vi "Step_Delay_Tommaso_fixed_EPICS.vi"() -> ()   [LabVIEW 2019]
uses:
  <vilib>/DAQmx/write.llb/DAQmx Write (Analog DBL 1Chan 1Samp).vi
  <vilib>/DAQmx/miscellaneous.llb/DAQmx Fill In Error Info.vi
  <vilib>/DAQmx/create/channels.llb/DAQmx Create Channel (AO-Voltage-Basic).vi
  <userlib>/caLab/Private/Put_Boolean-1D_PV.vi
  <vilib>/Analysis/1siggen.llb/Ramp Pattern by Delta.vi
  <userlib>/caLab/Private/Put_Boolean-1D_PV-1D.vi
  Driver/Newport ESP301/Newport ESP301.lvlib
  <vilib>/Analysis/NI_AALBase.lvlib
panel:
  out "IOC started":bool=TRUE
  in  "Config File":path=path "T:/trARPES/Labview/Front ends/METIS_delayscan/delayScanEPICS.conf" caption="Soft IOC configuration file"
  in  "Configuration Set":T1(array[cluster])=[{"PV name"="trARPES:DelayStage:t0", "description"="Delay Stage time zero Position", "data type"="ai", "number of elements (waveform only)"=1, "element size (waveform only)"="", []}, {"PV name"="trARPES:DelayStage:p1", "description"="Delay Stage range start", "data type"="ai", "number of elements (waveform only)"=1, "element size (waveform only)"="", []}, {"PV name"="trARPES:DelayStage:p2", "description"="Delay Stage range end", "data type"="ai", "number of elements (waveform only)"=1, "element size (waveform only)"="", []}, {"PV name"="trARPES:DelayStage:Pos", "description"="Current Delay Stage position", "data type"="ai", "number of elements (waveform only)"=1, "element size (waveform only)"="", []}]
  in  "Dwell_positions":string[][](table)=[["-500", "3000"], ["-100", "3000"], ["0", "5000"], ["100", "5000"], ["500", "5000"], ["750", "10000"], ["1000", "10000"], ["", ""]]
  in  "Enable2":bool caption="Enable?"
  in  "Wait time [ms]":u32=1000 caption="Values <50 \nwon't work"
  out "StepSize [mm]":dbl=0.14989622900000002
  in  "stop 2":bool
  in  "StepSize [fs]":i32=1000
  in  "Enable?":bool
  out "a":waveform(dbl)(graph)={"t0"=timestamp(3675940489.011235 s since 1904-01-01), "dt"=1.0, "Y"=[-33.8895]}
  out "Waveform Chart":dbl(graph)=5.25341140860948
  out "x*y":dbl=-876.4751437142558
  in  "physical channels":tag="Dev1/ao1"
  out "DAC error":errorcluster
  out "ESP error":errorcluster
  out "run?":bool
  in  "set_vel":bool
  in  "velocity [fs/s]":dbl=333.564095198152
  in  "vel_mm":dbl=0.005 caption="velocity [mm/s]"
  out "meas. velocity":dbl
  in  "stop":bool
  out "output voltage":dbl
  in  "start":bool
  in  "go2p1":bool
  out "position [mm]":dbl=-33.8895
  in  "p2 [mm]":dbl=-0.707153771
  in  "p1 [mm]":dbl=-1.006946229
  in  "interpolate output":bool
  in  "Delta2 [fs]":dbl=999.9999999999999
  in  "Delta1 [fs]":dbl=-999.9999999999999
  in  "Reference [mm]":dbl=-0.85705
  in  "Axis (1)":i32=3 min=1 max=3
  in  "Serial Link (RS232)":enum16{"RS232", "USB"}(ring)
  in  "VISA resource name":refnum<visa-resource-name>="COM8"
  in  "main_close":bool
  # "Interface panel"
  # "Velocity panel"
  # "Positions panel"
  # "Equally spaced steps panel"
  # "Controls panel"
  # "User-defined steps panel"
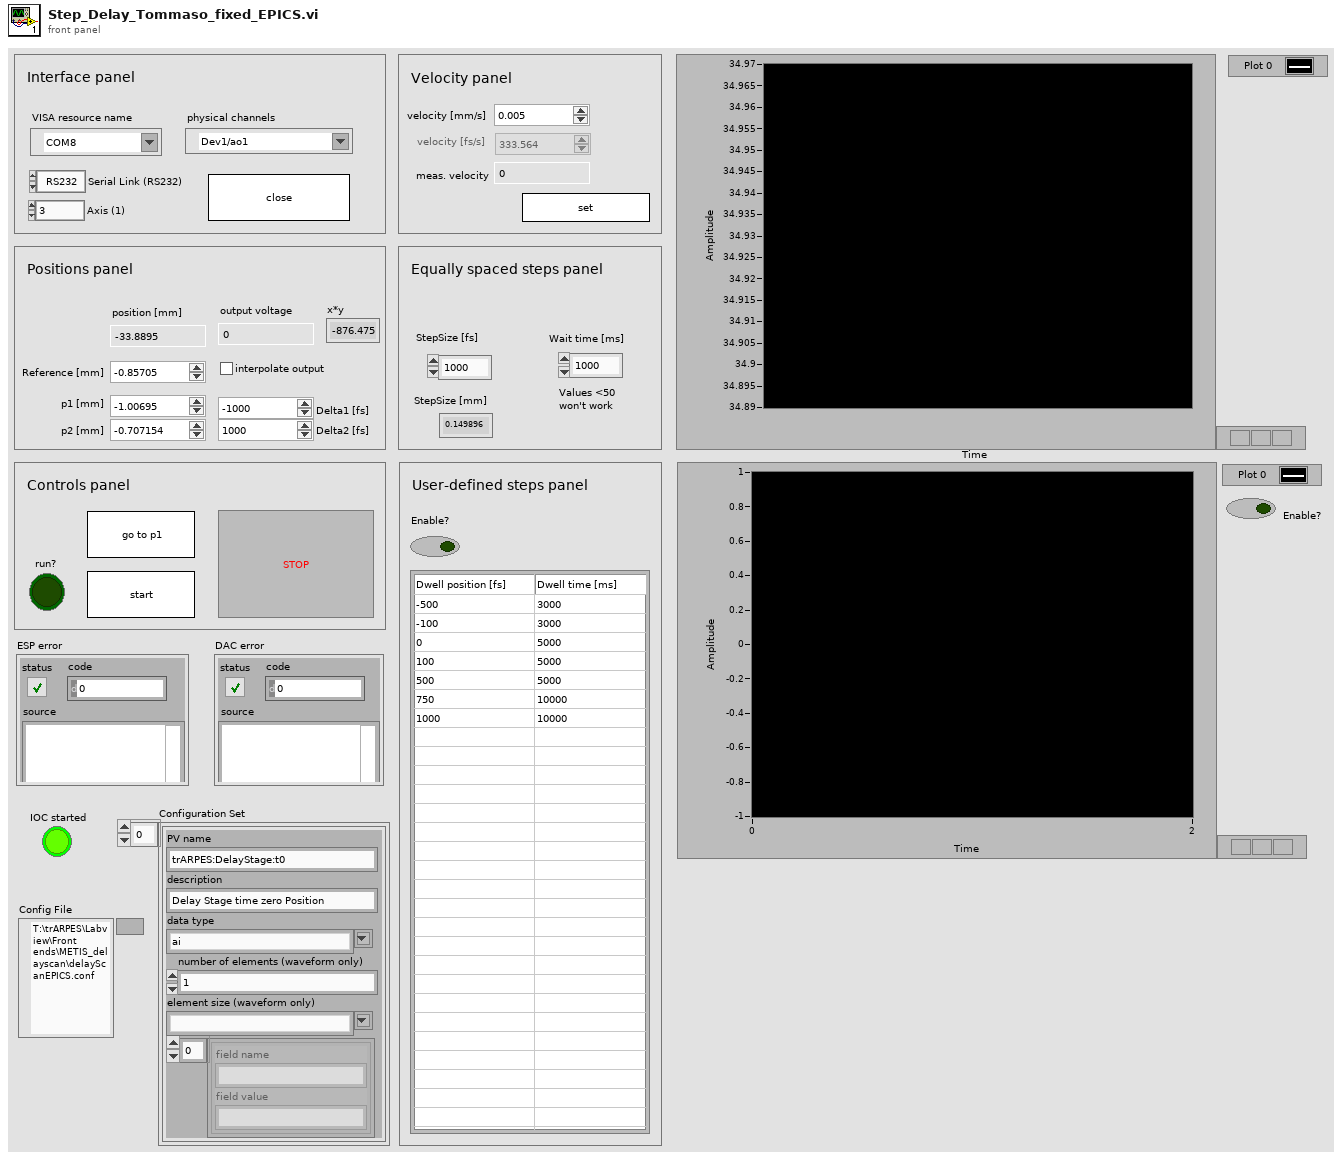
[diagram p1: front panel]
types:
  T1 = cluster{"PV name":string, "description":string, "data type":string, "number of elements (waveform only)":i32, "element size (waveform only)":string, cluster{"field name":string, "field value":string}[]}[]
  T2 = cluster{"dev1_data":refnum<queue>, "dev2_data":refnum<queue>}
  T3 = cluster{"dev1_cmd":refnum<queue>, "dev2_cmd":refnum<queue>}
  T4 = cluster{"PV Name":string, "Data Type":string, "Fields":cluster{"Field Name":string, "Field Value":string}[]}[]
  T5 = cluster{"PV Name":string, "Data Type":string, "Fields":cluster{"Field Name":string, "Field Value":string}[]}
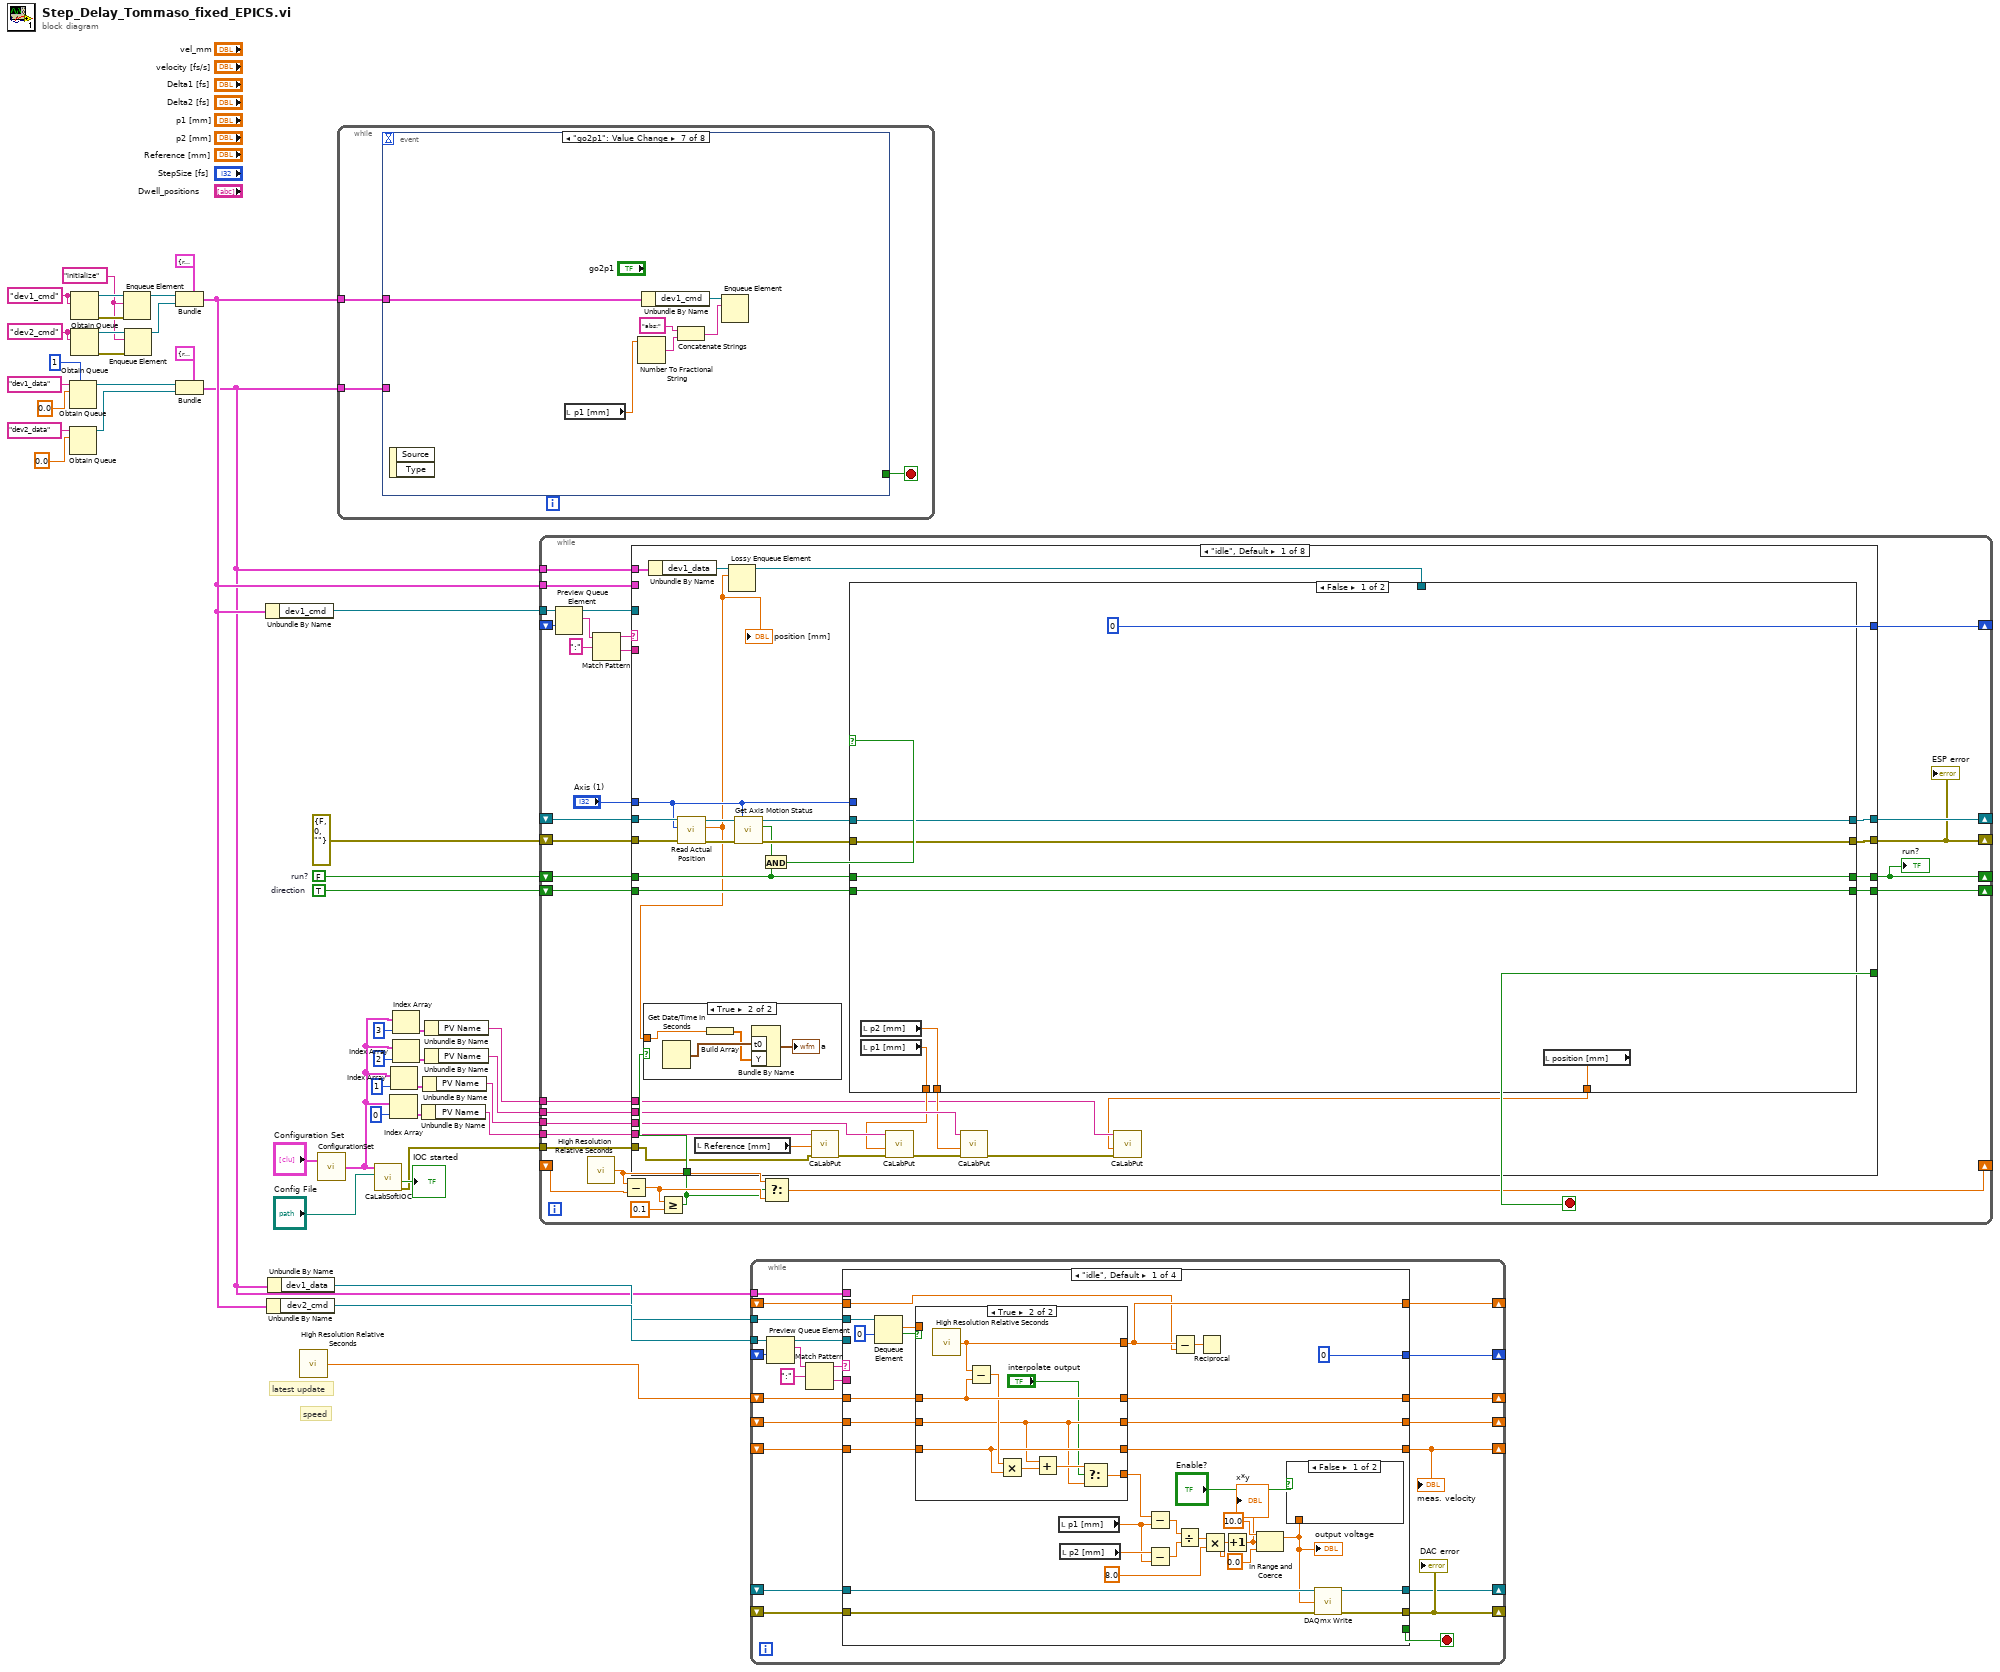
[diagram p0: block diagram]
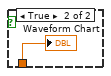
[diagram p2: hidden frame]
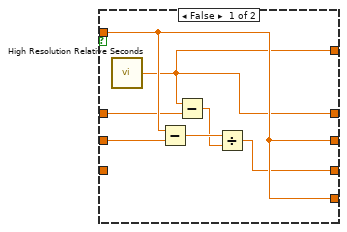
[diagram p3: hidden frame]
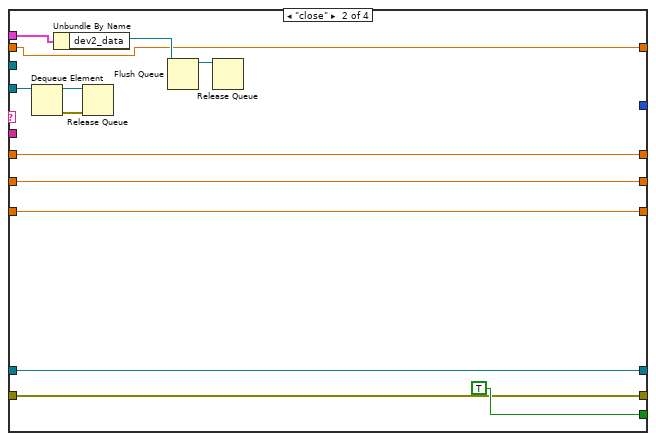
[diagram p4: hidden frame]
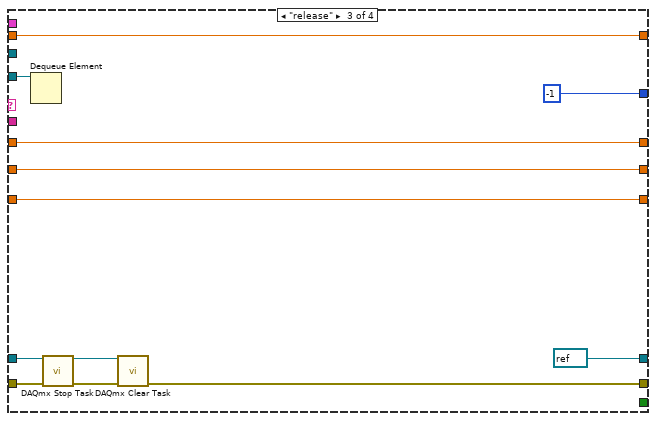
[diagram p5: hidden frame]
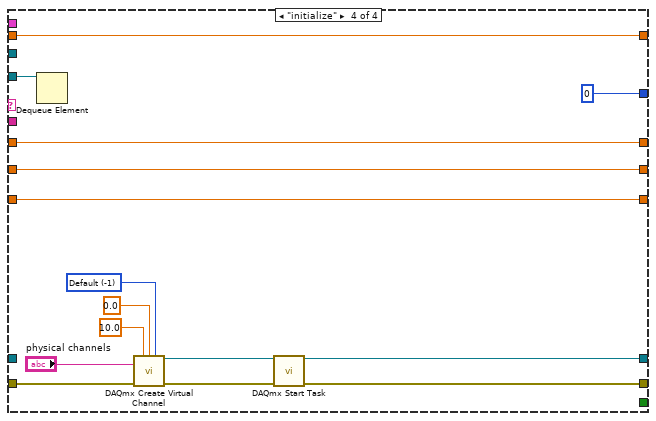
[diagram p6: hidden frame]
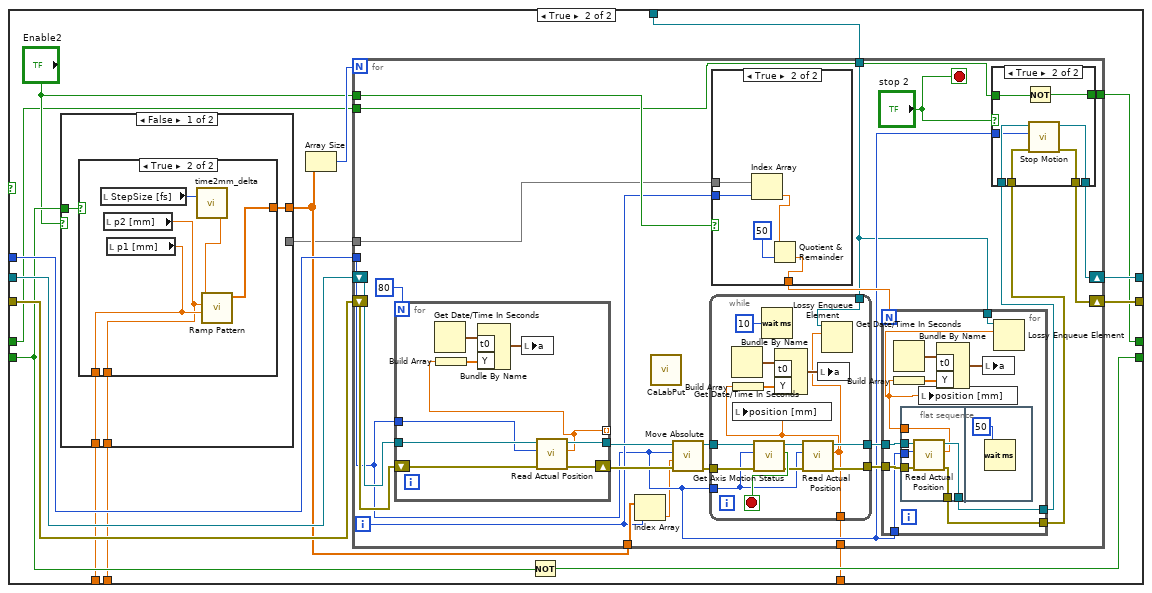
[diagram p8: hidden frame]
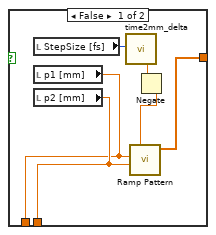
[diagram p9: hidden frame]
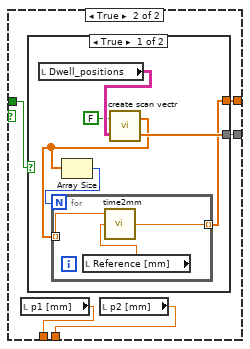
[diagram p10: hidden frame]
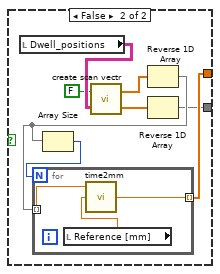
[diagram p11: hidden frame]
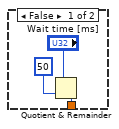
[diagram p13: hidden frame]
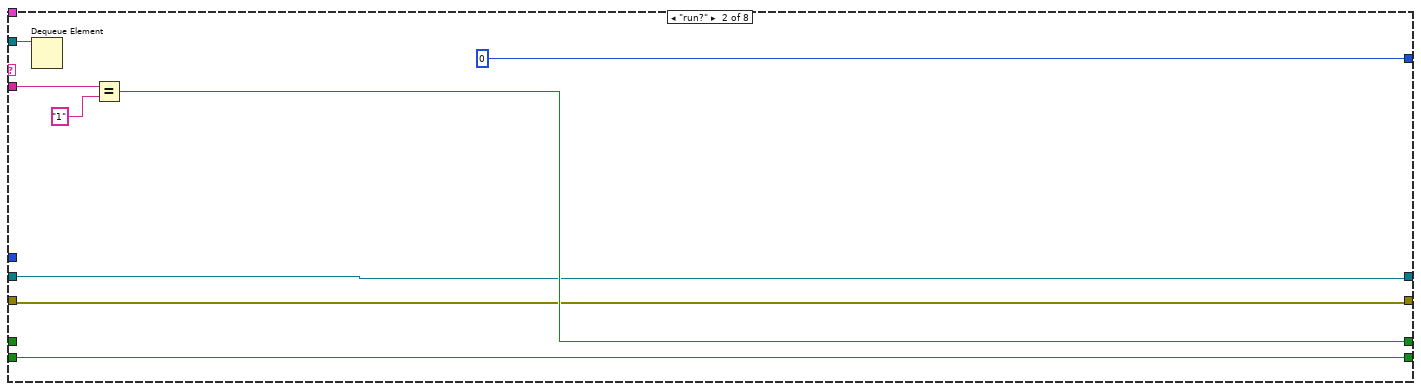
[diagram p14: hidden frame]
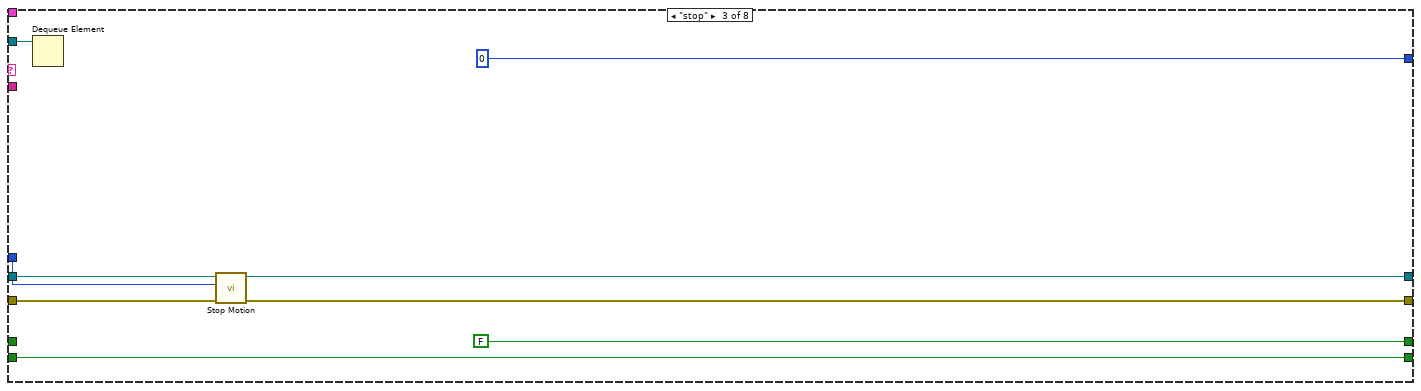
[diagram p15: hidden frame]
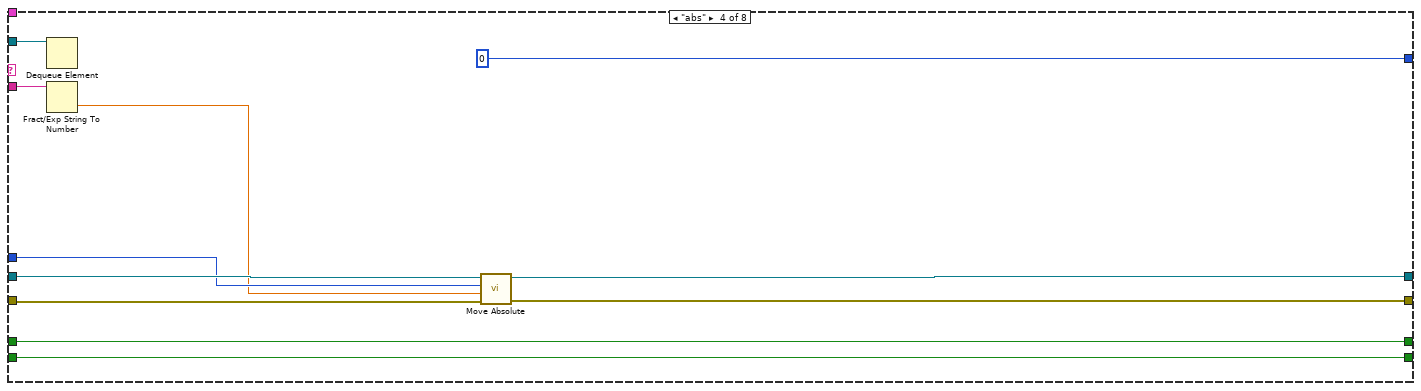
[diagram p16: hidden frame]
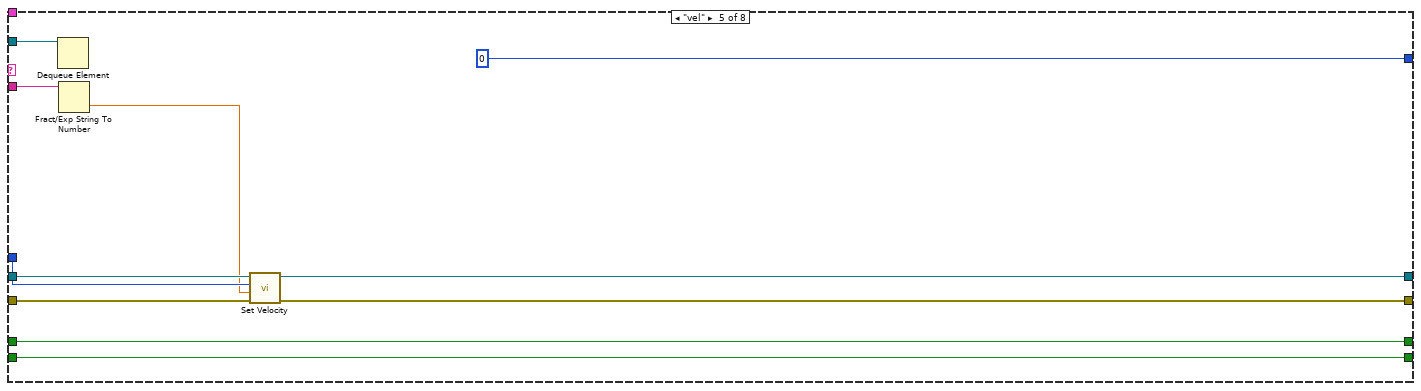
[diagram p17: hidden frame]
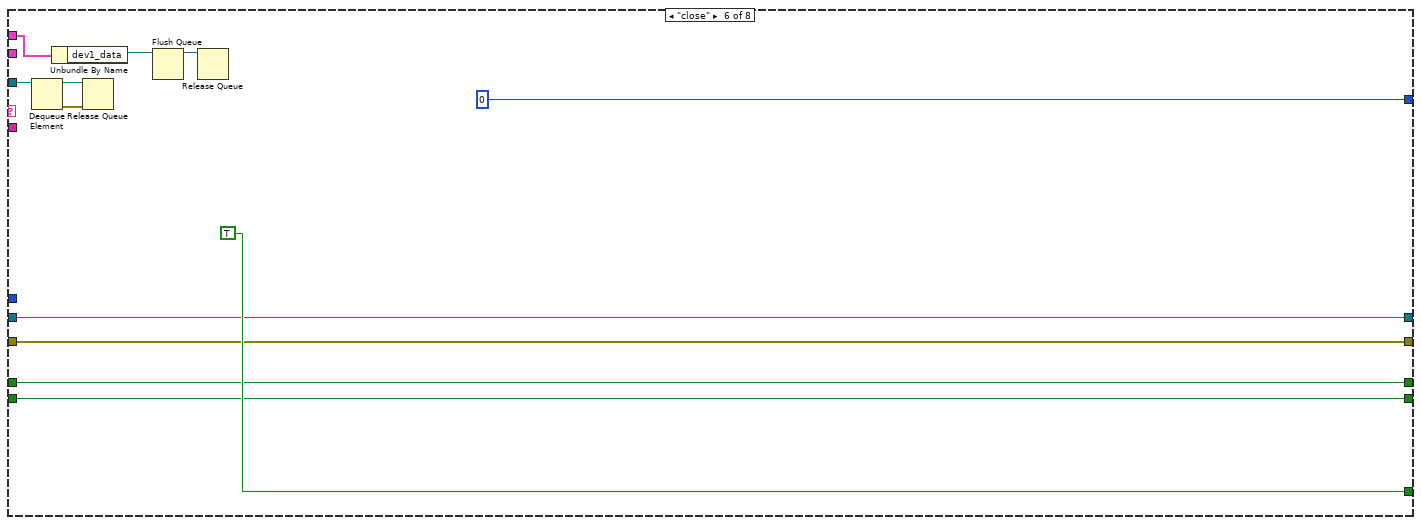
[diagram p18: hidden frame]
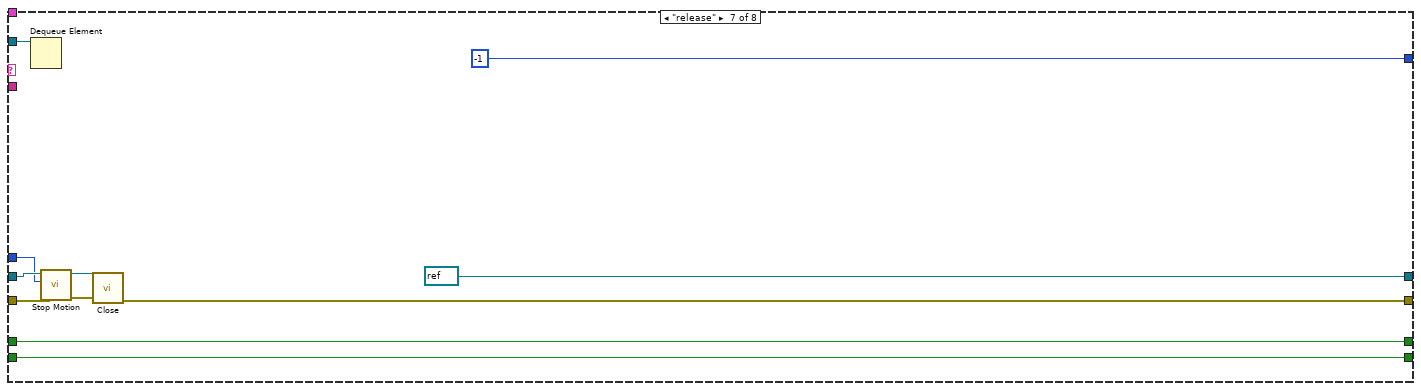
[diagram p19: hidden frame]
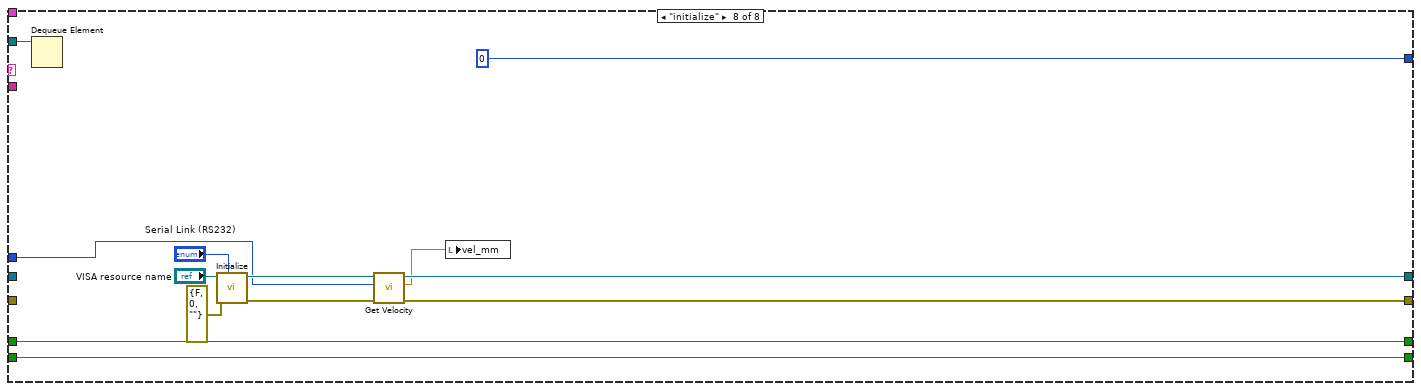
[diagram p20: hidden frame]
diagram:
  w18 = TRUE  # direction
  w21 = FALSE  # run?
  w32 = "dev2_cmd" ("name (unnamed)")
  w38 = "initialize" ("element")
  w33 = "dev1_cmd" ("name (unnamed)")
  # "speed"
  # "latest update"
  n1 = Obtain Queue(max queue size (-1, unlimited)=1, name (unnamed)="dev1_data", element data type=0.0) -> (queue out=w29:refnum<queue>)  [unwired: 2 in, 2 out]
  n2 = Obtain Queue(name (unnamed)="dev2_data", element data type=0.0) -> (queue out=w28:refnum<queue>)  [unwired: 3 in, 2 out]
  n3 = Obtain Queue(name (unnamed)=w33, element data type=w33) -> (queue out=w44:refnum<queue>, error out=w43:errorcluster)  [unwired: 3 in, 1 out]
  n4 = Obtain Queue(name (unnamed)=w32, element data type=w32) -> (queue out=w39:refnum<queue>, error out=w40:errorcluster)  [unwired: 3 in, 1 out]
  n5 = Enqueue Element(queue=w44, element=w38, error in (no error)=w43) -> (queue out=w41:refnum<queue>)  [unwired: 1 in, 2 out]
  n6 = Enqueue Element(queue=w39, element=w38, error in (no error)=w40) -> (queue out=w37:refnum<queue>)  [unwired: 1 in, 2 out]
  n7 = Bundle(cluster=T3 {"dev1_cmd"=refnum, "dev2_cmd"=refnum}, "dev1_cmd"=w41, "dev2_cmd"=w37) -> (w25:T3)
  n8 = Bundle(cluster=T2 {"dev1_data"=refnum, "dev2_data"=refnum}, "dev1_data"=w29, "dev2_data"=w28) -> (w19:T2)
  n9 = Unbundle By Name(w25) -> ("dev1_cmd"=w34:refnum<queue>)
  n10 = Unbundle By Name(w25) -> ("dev2_cmd"=w24:refnum<queue>)
  n11 = Unbundle By Name(w19) -> ("dev1_data"=w23:refnum<queue>)
  n12 = call <vilib>:"High Resolution Relative Seconds.vi"() -> ("relative seconds"=w22:dbl)
  n13 = call <userlib>:"ConfigurationSet.vi"("Configuration Set"="Configuration Set") -> ("PV set"=w7:T4)  [unwired: 1 in]
  n14 = while {
    tunnel: w25 -> [w47]
    tunnel: w19 -> [w46]
    stop <- w45 stop-if-true
    n15 = event shown="[6] \"go2p1\": Value Change" {
      selector: _ -> [_ _ _ _ _ _ _ _]
      dyn-events: _ -> [_ _ _ _ _ _ _ _]
      timeout: _ -> [_ _ _ _ _ _ _ _]
      tunnel: w47 -> [_ w51 _ _ w63 _ w81 w84]
      tunnel: w46 -> [_ _ _ _ _ _ _ _]
      tunnel: [_ _ _ _ _ _ _ TRUE] -> w45
      event Timeout {
        n16 = event-data() -> ()  [unwired: 1 in, 1 out]
      }
      event "start", "stop": Value Change {
        n17 = event-data() -> ()  [unwired: 1 in, 1 out]
        n18 = Boolean To (0,1)(Boolean="start") -> (0, 1=w49:i16)
        n19 = Number To Decimal String(number=w49) -> (decimal integer string=w48:string)  [unwired: 1 in]
        n20 = Unbundle By Name(w51) -> ("dev1_cmd"=w54:refnum<queue>)
        n21 = Concatenate Strings("run?:" ("string"), w48) -> (w53:string)
        n22 = Enqueue Element(queue=w54, element=w53) -> ()  [unwired: 2 in, 3 out]
      }
      event "StepSize [fs]": Value Change {
        n23 = event-data() -> ("NewVal"=w55:i32)  [unwired: 1 in, 5 out]
        n24 = call "time2mm_delta.vi"("Delta time"=w55) -> ("Delta position (mm)"=→"StepSize [mm]":dbl)  [unwired: 2 in]
      }
      event "Delta1 [fs]", "Delta2 [fs]": Value Change {
        n25 = event-data() -> ()  [unwired: 1 in, 1 out]
        n26 = local read "Reference [mm]"() -> (w58:dbl)
        n27 = local read "Delta2 [fs]"() -> (w59:dbl)
        n28 = local read "Delta1 [fs]"() -> (w61:dbl)
        n29 = call "time2mm.vi"("Offset (mm)"=w58, "time"=w61) -> ("position (mm)"=w60:dbl)  [unwired: 1 in]
        n30 = call "time2mm.vi"("Offset (mm)"=w58, "time"=w59) -> ("position (mm)"=w57:dbl)  [unwired: 1 in]
        n31 = local write "p2 [mm]"(w57) -> ()
        n32 = local write "p1 [mm]"(w60) -> ()
      }
      event "set_vel": Value Change {
        n33 = event-data() -> ()  [unwired: 1 in, 2 out]
        n34 = local read "vel_mm"() -> (w62:dbl)
        n35 = Number To Fractional String(number=w62) -> (F-format string=w66:string)  [unwired: 3 in]
        n36 = Unbundle By Name(w63) -> ("dev1_cmd"=w67:refnum<queue>)
        n37 = Concatenate Strings("vel:" ("string"), w66) -> (w65:string)
        n38 = Enqueue Element(queue=w67, element=w65) -> ()  [unwired: 2 in, 3 out]
      }
      event "p1 [mm]", "p2 [mm]", "Reference [mm]", "vel_mm": Value Change {
        n39 = event-data() -> ()  [unwired: 1 in, 2 out]
        n40 = local read "Reference [mm]"() -> (w73:dbl)
        n41 = local read "vel_mm"() -> (w70:dbl)
        n42 = local read "p1 [mm]"() -> (w74:dbl)
        n43 = local read "p2 [mm]"() -> (w75:dbl)
        n44 = call "mm2time.vi"("Offset (mm)"=0.0, "distance (mm)"=w70) -> ("time in fs"=w69:dbl)  [unwired: 1 in]
        n45 = call "mm2time.vi"("Offset (mm)"=w73, "distance (mm)"=w74) -> ("time in fs"=w71:dbl)  [unwired: 1 in]
        n46 = call "mm2time.vi"("Offset (mm)"=w73, "distance (mm)"=w75) -> ("time in fs"=w72:dbl)  [unwired: 1 in]
        n47 = local write "velocity [fs/s]"(w69) -> ()
        n48 = local write "Delta1 [fs]"(w71) -> ()
        n49 = local write "Delta2 [fs]"(w72) -> ()
      }
      event "go2p1": Value Change {
        n50 = event-data() -> ()  [unwired: 1 in, 2 out]
        n51 = local read "p1 [mm]"() -> (w76:dbl)
        n52 = Number To Fractional String(number=w76) -> (F-format string=w79:string)  [unwired: 3 in]
        n53 = Unbundle By Name(w81) -> ("dev1_cmd"=w80:refnum<queue>)
        n54 = Concatenate Strings("abs:" ("string"), w79) -> (w77:string)
        n55 = Enqueue Element(queue=w80, element=w77) -> ()  [unwired: 2 in, 3 out]
      }
      event "main_close": Value Change {
        n56 = event-data() -> ()  [unwired: 1 in, 1 out]
        n57 = Cluster To Array(cluster=w84) -> (array=w83:refnum<queue>[])
        n58 = for {
          tunnel: w83 -> [w89] mode=indexing
          n59 = Flush Queue(queue=w89) -> (queue out=w85:refnum<queue>)  [unwired: 1 in, 2 out]
          n60 = Enqueue Element(queue=w85, element="release") -> (queue out=w87:refnum<queue>)  [unwired: 2 in, 2 out]
          n61 = Enqueue Element(queue=w87, element="close") -> ()  [unwired: 2 in, 3 out]
        }
      }
    }
  }
  n62 = call <userlib>:"CaLabSoftIOC.vi"("Config File"="Config File", "PV set"=w7) -> ("error out"=w5:errorcluster, "IOC started"=→"IOC started":bool)  [unwired: 4 in, 2 out]
  n63 = Index Array(array=w7, index=0) -> (element=w16:T5)
  n64 = Index Array(array=w7, index=1) -> (element=w12:T5)
  n65 = Index Array(array=w7, index=3) -> (element=w8:T5)
  n66 = Index Array(array=w7, index=2) -> (element=w11:T5)
  n67 = Unbundle By Name(w16) -> ("PV Name"=w4:string)
  n68 = Unbundle By Name(w12) -> ("PV Name"=w3:string)
  n69 = Unbundle By Name(w8) -> ("PV Name"=w1:string)
  n70 = Unbundle By Name(w11) -> ("PV Name"=w2:string)
  n71 = while {
    tunnel: w25 -> [w115]
    tunnel: w34 -> [w120]
    tunnel: w19 -> [w112]
    shift-right: [w110] -> _
    shift-left: _ -> [w111]
    shift-right: [w109] -> _
    shift-left: _ -> [w106]
    shift-right: [w108] -> _
    shift-left: errorcluster {"status"=FALSE, "code"=0, "source"=""} ("error out") -> [w107]
    shift-right: [w103] -> _
    shift-left: w21 -> [w104]
    shift-right: [w101] -> _
    shift-left: w18 -> [w102]
    shift-right: [w95] -> _
    shift-left: _ -> [w100]
    tunnel: w5 -> [w94]
    tunnel: w4 -> [w93]
    tunnel: w3 -> [w92]
    tunnel: w2 -> [w91]
    tunnel: w1 -> [w90]
    stop <- w113 stop-if-true
    n72 = Preview Queue Element(queue=w120, timeout in ms (-1)=w111) -> (queue out=w114:refnum<queue>, element=w119:string)  [unwired: 1 in, 2 out]
    n73 = call <vilib>:"High Resolution Relative Seconds.vi"() -> ("relative seconds"=w97:dbl)
    n74 = Match Pattern(string=w119, regular expression=":") -> (before substring=w117:string, after substring=w116:string)  [unwired: 1 in, 2 out]
    n75 = Subtract(x=w97, y=w100) -> (x-y=w98:dbl)
    n76 = Greater Or Equal?(x=w98, y=0.1) -> (x >= y?=w96:bool)
    n77 = case shown="\"idle\", Default" w117 {
      tunnel: w116 -> [_ w312 _ w331 w338 _ _ _]
      tunnel: w115 -> [_ _ _ _ _ _ _ _]
      tunnel: w114 -> [_ w310 w314 w332 w336 w355 w365 w375]
      tunnel: [_ _ _ _ _ TRUE _ _] -> w113
      tunnel: w112 -> [w152 _ _ _ _ w347 _ _]
      tunnel: [0 0 0 0 0 0 -1 0] -> w110
      tunnel: [w150 w305 w319 w328 w343 w351 refnum<visa-resource-name> refnum ("VISA resource name out") w371] -> w109
      tunnel: [w149 w306 w318 w327 w342 w350 w364 w370] -> w108
      tunnel: w107 -> [w147 w306 w320 w329 w341 w350 w360 _]
      tunnel: w106 -> [w148 w305 w321 w330 w340 w351 w357 _]
      tunnel: "Axis (1)" -> [w138 _ w317 w326 w339 _ w356 w372]
      tunnel: w104 -> [w136 _ _ w323 w334 w348 w362 w376]
      tunnel: [w144 w308 FALSE ("run?") w323 w334 w348 w362 w376] -> w103
      tunnel: w102 -> [w145 w307 w313 w322 w333 w344 w361 w367]
      tunnel: [w146 w307 w313 w322 w333 w344 w361 w367] -> w101
      tunnel: w96 -> [w134 _ _ _ _ _ _ _]
      tunnel: w94 -> [w125 _ _ _ _ _ _ _]
      tunnel: w93 -> [w133 _ _ _ _ _ _ _]
      tunnel: w92 -> [w132 _ _ _ _ _ _ _]
      tunnel: w91 -> [w131 _ _ _ _ _ _ _]
      tunnel: w90 -> [w123 _ _ _ _ _ _ _]
      frame "idle", Default {
        n78 = Unbundle By Name(w152) -> ("dev1_data"=w151:refnum<queue>)
        n79 = call "Read Actual Position.vi"("error in (no error)"=w147, "Axis (1)"=w138, "VISA resource name"=w148) -> ("error out"=w141:errorcluster, "Position (units)"=w128:dbl, "VISA resource name out"=w142:refnum<visa-resource-name>)  [unwired: 2 in]
        "position [mm]" <- w128
        n80 = case shown="True" w134 {
          tunnel: w128 -> [_ w157]
          frame False {
          }
          frame True {
            n81 = Get Date/Time In Seconds() -> (seconds since 1Jan1904=w156:timestamp)
            n82 = Build Array(w157) -> (w155:dbl[])
            n83 = Bundle By Name("t0"=w156, "Y"=w155) -> (→"a":waveform(dbl))  [unwired: 1 in]
          }
        }
        n84 = local read "Reference [mm]"() -> (w124:dbl)
        n85 = Lossy Enqueue Element(queue=w151, element=w128) -> (queue out=w143:refnum<queue>)  [unwired: 1 in, 3 out]
        n86 = call "Get Axis Motion Status.vi"("error in (no error)"=w141, "Axis (1)"=w138, "VISA resource name"=w142) -> ("error out"=w139:errorcluster, "Motion Done"=w137:bool, "VISA resource name out"=w140:refnum<visa-resource-name>)  [unwired: 2 in]
        n87 = And(x=w137, y=w136) -> (x .and. y?=w135:bool)
        n88 = call-poly <userlib>:"CaLabPut.vi"("Error in (no error)"=w125, "Timeout (3)"=w124, "PV Name"=w133) -> ("Error out"=w130:errorcluster)  [unwired: 5 in, 3 out]
        n89 = case shown="False" w135 {
          tunnel: w140 -> [w164 w180]
          tunnel: w139 -> [w163 w181]
          tunnel: [w164 w179] -> w150
          tunnel: [w163 w178] -> w149
          tunnel: w138 -> [_ w177]
          tunnel: [w162 w176] -> w146
          tunnel: w145 -> [w162 w175]
          tunnel: w136 -> [w161 w170]
          tunnel: [w161 w169] -> w144
          tunnel: w143 -> [_ w168]
          tunnel: [w160 w167] -> w127
          tunnel: [w159 w166] -> w126
          tunnel: [w158 w165] -> w121
          frame False {
            n90 = local read "p2 [mm]"() -> (w159:dbl)
            n91 = local read "p1 [mm]"() -> (w160:dbl)
            n92 = local read "position [mm]"() -> (w158:dbl)
          }
          frame True {
            n93 = case shown="False" "Enable2" {
              tunnel: w175 -> [w185 w199]
              tunnel: [w184 w200] -> w174
              tunnel: [_ w201] -> w171
              tunnel: [w183 w198] -> w167
              tunnel: [w182 w197] -> w166
              frame False {
                n94 = case shown="True" w185 {
                  tunnel: [w191 w196] -> w184
                  tunnel: [w186 w193] -> w183
                  tunnel: [w187 w192] -> w182
                  frame False {
                    n95 = local read "StepSize [fs]"() -> (w188:i32)
                    n96 = local read "p1 [mm]"() -> (w186:dbl)
                    n97 = local read "p2 [mm]"() -> (w187:dbl)
                    n98 = call "time2mm_delta.vi"("Delta time"=w188) -> ("Delta position (mm)"=w189:dbl)  [unwired: 2 in]
                    n99 = Negate(x=w189) -> (-x=w190:dbl)
                    n100 = call-poly <vilib>:"Ramp Pattern.vi"("start"=w187, "end"=w186, "delta"=w190) -> ("Ramp Pattern"=w191:dbl[])  [unwired: 6 in, 2 out]
                  }
                  frame True {
                    n101 = local read "StepSize [fs]"() -> (w194:i32)
                    n102 = local read "p2 [mm]"() -> (w192:dbl)
                    n103 = local read "p1 [mm]"() -> (w193:dbl)
                    n104 = call "time2mm_delta.vi"("Delta time"=w194) -> ("Delta position (mm)"=w195:dbl)  [unwired: 2 in]
                    n105 = call-poly <vilib>:"Ramp Pattern.vi"("start"=w193, "end"=w192, "delta"=w195) -> ("Ramp Pattern"=w196:dbl[])  [unwired: 6 in, 2 out]
                  }
                }
              }
              frame True {
                n106 = local read "p1 [mm]"() -> (w198:dbl)
                n107 = case shown="True" w199 {
                  tunnel: [w205 w211] -> w201
                  tunnel: [w204 w216] -> w200
                  frame True {
                    n108 = local read "Dwell_positions"() -> (w207:string[][])
                    n109 = call "create scan vectr.vi"("Table Control"=w207, "waypoint mode?"=FALSE) -> ("Array 2"=w205:dbl[], "Array"=w203:dbl[])
                    n110 = Array Size(array=w203) -> (size(s)=w202:i32)
                    n111 = for {
                      N: w202 -> [_]
                      tunnel: w203 -> [w210] mode=indexing
                      tunnel: [w209] -> w204 mode=indexing
                      n112 = local read "Reference [mm]"() -> (w208:dbl)
                      n113 = call "time2mm.vi"("Offset (mm)"=w208, "time"=w210) -> ("position (mm)"=w209:dbl)  [unwired: 1 in]
                    }
                  }
                  frame False {
                    n114 = local read "Dwell_positions"() -> (w218:string[][])
                    n115 = call "create scan vectr.vi"("Table Control"=w218, "waypoint mode?"=FALSE) -> ("Array 2"=w212:dbl[], "Array"=w213:dbl[])
                    n116 = Reverse 1D Array(array=w213) -> (reversed array=w214:dbl[])
                    n117 = Array Size(array=w214) -> (size(s)=w215:i32)
                    n118 = for {
                      N: w215 -> [_]
                      tunnel: w214 -> [w221] mode=indexing
                      tunnel: [w220] -> w216 mode=indexing
                      n119 = local read "Reference [mm]"() -> (w219:dbl)
                      n120 = call "time2mm.vi"("Offset (mm)"=w219, "time"=w221) -> ("position (mm)"=w220:dbl)  [unwired: 1 in]
                    }
                    n121 = Reverse 1D Array(array=w212) -> (reversed array=w211:dbl[])
                  }
                }
                n122 = local read "p2 [mm]"() -> (w197:dbl)
              }
            }
            n123 = Array Size(array=w174) -> (size(s)=w173:i32)
            n124 = for {
              N: w173 -> [_]
              tunnel: w177 -> [w227]
              tunnel: w174 -> [w242]
              shift-right: [w229] -> w178
              shift-left: w181 -> [w245]
              shift-right: [w231] -> w179
              shift-left: w180 -> [w244]
              tunnel: "Enable2" -> [w235]
              tunnel: w171 -> [w233]
              tunnel: w170 -> [w226]
              tunnel: [w225] -> w169
              tunnel: w168 -> [w224]
              tunnel: [w222] -> w165
              i -> [w234]
              stop <- "stop 2" stop-if-true
              n125 = for {
                N: 80 -> [_]
                tunnel: w244 -> [w304]
                tunnel: [w303] -> w243
                shift-right: [w300] -> w239
                shift-left: w245 -> [w302]
                tunnel: w227 -> [w301]
                tunnel: [w297] -> _ mode=indexing
                n126 = Get Date/Time In Seconds() -> (seconds since 1Jan1904=w298:timestamp)
                n127 = call "Read Actual Position.vi"("error in (no error)"=w302, "Axis (1)"=w301, "VISA resource name"=w304) -> ("error out"=w300:errorcluster, "Position (units)"=w297:dbl, "VISA resource name out"=w303:refnum<visa-resource-name>)  [unwired: 2 in]
                n128 = Build Array(w297) -> (w299:dbl[])
                n129 = Bundle By Name("t0"=w298, "Y"=w299) -> (w296:waveform(dbl))  [unwired: 1 in]
                n130 = local write "a"(w296) -> ()
              }
              n131 = Index Array(array=w242, index=w234) -> (element=w223:dbl)
              n132 = call-poly <userlib>:"CaLabPut.vi"() -> ()  [unwired: 8 in, 4 out]
              n133 = call "Move Absolute.vi"("error in (no error)"=w239, "Position (0 units)"=w223, "Axis (1)"=w227, "VISA resource name"=w243) -> ("error out"=w240:errorcluster, "VISA resource name out"=w241:refnum<visa-resource-name>)  [unwired: 2 in]
              n134 = while {
                tunnel: w241 -> [w295]
                tunnel: [w290] -> w236
                tunnel: w240 -> [w294]
                tunnel: [w288] -> w237
                tunnel: w227 -> [w287]
                tunnel: w224 -> [w283]
                tunnel: [w282] -> w222
                stop <- w292 stop-if-true
                n135 = Get Date/Time In Seconds() -> (seconds since 1Jan1904=w286:timestamp)
                n136 = call "Get Axis Motion Status.vi"("error in (no error)"=w294, "Axis (1)"=w287, "VISA resource name"=w295) -> ("error out"=w289:errorcluster, "Motion Done"=w292:bool, "VISA resource name out"=w291:refnum<visa-resource-name>)  [unwired: 2 in]
                n137 = Wait (ms)(milliseconds to wait=10) -> ()  [unwired: 1 out]
                n138 = call "Read Actual Position.vi"("error in (no error)"=w289, "Axis (1)"=w287, "VISA resource name"=w291) -> ("error out"=w288:errorcluster, "Position (units)"=w282:dbl, "VISA resource name out"=w290:refnum<visa-resource-name>)  [unwired: 2 in]
                n139 = Build Array(w282) -> (w285:dbl[])
                n140 = local write "position [mm]"(w282) -> ()
                n141 = Bundle By Name("t0"=w286, "Y"=w285) -> (w284:waveform(dbl))  [unwired: 1 in]
                n142 = local write "a"(w284) -> ()
                n143 = Lossy Enqueue Element(queue=w283, element=w282) -> ()  [unwired: 1 in, 4 out]
              }
              n144 = case shown="True" w235 {
                tunnel: [w257 w263] -> w238
                tunnel: w234 -> [_ w261]
                tunnel: w233 -> [_ w260]
                frame False {
                  n145 = Quotient & Remainder(x="Wait time [ms]", y=50) -> (floor(x/y)=w257:u32)  [unwired: 1 out]
                }
                frame True {
                  n146 = Index Array(array=w260, index=w261) -> (element=w262:dbl)
                  n147 = Quotient & Remainder(x=w262, y=50) -> (floor(x/y)=w263:dbl)  [unwired: 1 out]
                }
              }
              n148 = for {
                N: w238 -> [_]
                tunnel: w237 -> [w274]
                tunnel: [w273] -> w230
                tunnel: w236 -> [w272]
                tunnel: [w271] -> w232
                tunnel: w227 -> [w270]
                tunnel: w224 -> [w265]
                n149 = Get Date/Time In Seconds() -> (seconds since 1Jan1904=w268:timestamp)
                n150 = Build Array(w266) -> (w269:dbl[])
                n151 = flat-sequence {
                  tunnel: w274 -> [w280]
                  tunnel: [w279] -> w273
                  tunnel: w272 -> [w278]
                  tunnel: [w277] -> w271
                  tunnel: w270 -> [w276]
                  tunnel: [w275] -> w266
                  frame #0 {
                    n152 = call "Read Actual Position.vi"("error in (no error)"=w280, "Axis (1)"=w276, "VISA resource name"=w278) -> ("error out"=w279:errorcluster, "Position (units)"=w275:dbl, "VISA resource name out"=w277:refnum<visa-resource-name>)  [unwired: 2 in]
                  }
                  frame #1 {
                    n153 = Wait (ms)(milliseconds to wait=50) -> ()  [unwired: 1 out]
                  }
                }
                n154 = local write "position [mm]"(w266) -> ()
                n155 = Bundle By Name("t0"=w268, "Y"=w269) -> (w267:waveform(dbl))  [unwired: 1 in]
                n156 = local write "a"(w267) -> ()
                n157 = Lossy Enqueue Element(queue=w265, element=w266) -> ()  [unwired: 1 in, 4 out]
              }
              n158 = case shown="True" "stop 2" {
                tunnel: w232 -> [w249 w256]
                tunnel: [w249 w255] -> w231
                tunnel: w230 -> [w248 w254]
                tunnel: [w248 w253] -> w229
                tunnel: w227 -> [_ w252]
                tunnel: w226 -> [w247 w251]
                tunnel: [w247 w250] -> w225
                frame False {
                }
                frame True {
                  n159 = Not(x=w251) -> (.not. x?=w250:bool)
                  n160 = call "Stop Motion.vi"("error in (no error)"=w254, "Axis (1)"=w252, "VISA resource name"=w256) -> ("error out"=w253:errorcluster, "VISA resource name out"=w255:refnum<visa-resource-name>)  [unwired: 3 in]
                }
              }
            }
            n161 = Not(x=w175) -> (.not. x?=w176:bool)
          }
        }
        n162 = call-poly <userlib>:"CaLabPut.vi"("Error in (no error)"=w130, "Timeout (3)"=w127, "PV Name"=w132) -> ("Error out"=w129:errorcluster)  [unwired: 5 in, 3 out]
        n163 = call-poly <userlib>:"CaLabPut.vi"("Error in (no error)"=w129, "Timeout (3)"=w126, "PV Name"=w131) -> ("Error out"=w122:errorcluster)  [unwired: 5 in, 3 out]
        n164 = call-poly <userlib>:"CaLabPut.vi"("Error in (no error)"=w122, "Timeout (3)"=w121, "PV Name"=w123) -> ()  [unwired: 5 in, 4 out]
      }
      frame "run?" {
        n165 = Dequeue Element(queue=w310) -> ()  [unwired: 2 in, 4 out]
        n166 = Equal?(x=w312, y="1") -> (x = y?=w308:bool)
      }
      frame "stop" {
        n167 = Dequeue Element(queue=w314) -> ()  [unwired: 2 in, 4 out]
        n168 = call "Stop Motion.vi"("error in (no error)"=w320, "Axis (1)"=w317, "VISA resource name"=w321) -> ("error out"=w318:errorcluster, "VISA resource name out"=w319:refnum<visa-resource-name>)  [unwired: 3 in]
      }
      frame "abs" {
        n169 = Dequeue Element(queue=w332) -> ()  [unwired: 2 in, 4 out]
        n170 = Fract/Exp String To Number(string=w331) -> (number=w325:dbl)  [unwired: 3 in, 1 out]
        n171 = call "Move Absolute.vi"("error in (no error)"=w329, "Position (0 units)"=w325, "Axis (1)"=w326, "VISA resource name"=w330) -> ("error out"=w327:errorcluster, "VISA resource name out"=w328:refnum<visa-resource-name>)  [unwired: 2 in]
      }
      frame "vel" {
        n172 = Dequeue Element(queue=w336) -> ()  [unwired: 2 in, 4 out]
        n173 = Fract/Exp String To Number(string=w338) -> (number=w337:dbl)  [unwired: 3 in, 1 out]
        n174 = call "Set Velocity.vi"("error in (no error)"=w341, "Velocity (units/s)"=w337, "Axis (1)"=w339, "VISA resource name"=w340) -> ("error out"=w342:errorcluster, "VISA resource name out"=w343:refnum<visa-resource-name>)  [unwired: 2 in]
      }
      frame "close" {
        n175 = Dequeue Element(queue=w355) -> (queue out=w354:refnum<queue>, error out=w353:errorcluster)  [unwired: 2 in, 2 out]
        n176 = Unbundle By Name(w347) -> ("dev1_data"=w345:refnum<queue>)
        n177 = Release Queue(queue=w354, error in (no error)=w353) -> ()  [unwired: 1 in, 3 out]
        n178 = Flush Queue(queue=w345) -> (queue out=w346:refnum<queue>)  [unwired: 1 in, 2 out]
        n179 = Release Queue(queue=w346) -> ()  [unwired: 2 in, 3 out]
      }
      frame "release" {
        n180 = Dequeue Element(queue=w365) -> ()  [unwired: 2 in, 4 out]
        n181 = call "Stop Motion.vi"("error in (no error)"=w360, "Axis (1)"=w356, "VISA resource name"=w357) -> ("error out"=w359:errorcluster, "VISA resource name out"=w358:refnum<visa-resource-name>)  [unwired: 3 in]
        n182 = call "Close.vi"("error in (no error)"=w359, "VISA resource name"=w358) -> ("error out"=w364:errorcluster)  [unwired: 9 in]
      }
      frame "initialize" {
        n183 = Dequeue Element(queue=w375) -> ()  [unwired: 2 in, 4 out]
        n184 = call "Initialize.vi"("VISA resource name"="VISA resource name", "error in (no error)"=errorcluster {"status"=FALSE, "code"=0, "source"=""}, "Serial Link (RS232)"="Serial Link (RS232)") -> ("VISA resource name out"=w374:refnum<visa-resource-name>, "error out"=w373:errorcluster)  [unwired: 6 in]
        n185 = call "Get Velocity.vi"("error in (no error)"=w373, "Axis (1)"=w372, "VISA resource name"=w374) -> ("error out"=w370:errorcluster, "Velocity (units/s)"=w369:dbl, "VISA resource name out"=w371:refnum<visa-resource-name>)  [unwired: 2 in]
        n186 = local write "vel_mm"(w369) -> ()
      }
    }
    "run?" <- w103
    "ESP error" <- w108
    n187 = Select(t=w97, s=w96, f=w98) -> (s? t:f=w95:dbl)
  }
  n188 = while {
    shift-right: [w395] -> _
    shift-left: _ -> [w396]
    shift-right: [w394] -> _
    shift-left: _ -> [w393]
    tunnel: w24 -> [w392]
    shift-right: [w391] -> _
    shift-left: _ -> [w390]
    tunnel: w23 -> [w389]
    shift-right: [w388] -> _
    shift-left: _ -> [w385]
    shift-right: [w387] -> _
    shift-left: w22 -> [w386]
    shift-right: [w380] -> _
    shift-left: _ -> [w384]
    tunnel: w19 -> [w383]
    shift-right: [w382] -> _
    shift-left: _ -> [w381]
    stop <- w397 stop-if-true
    n189 = Preview Queue Element(queue=w392, timeout in ms (-1)=w396) -> (queue out=w398:refnum<queue>, element=w402:string)  [unwired: 1 in, 2 out]
    n190 = Match Pattern(string=w402, regular expression=":") -> (before substring=w400:string, after substring=w399:string)  [unwired: 1 in, 2 out]
    n191 = case shown="\"idle\", Default" w400 {
      tunnel: w399 -> [_ _ _ _]
      tunnel: w398 -> [_ w463 w474 w482]
      tunnel: [_ TRUE _ _] -> w397
      tunnel: [0 _ -1 0] -> w395
      tunnel: [w429 w459 w473 w483] -> w394
      tunnel: w393 -> [w427 w459 w470 w490]
      tunnel: [w430 w458 refnum<k21> refnum ("task out") w484] -> w391
      tunnel: w390 -> [w428 w458 w471 _]
      tunnel: w389 -> [w431 _ _ _]
      tunnel: [w425 w456 w466 w479] -> w388
      tunnel: [w424 w457 w467 w480] -> w387
      tunnel: w386 -> [w422 w457 w467 w480]
      tunnel: w385 -> [w423 w456 w466 w479]
      tunnel: [w421 w455 w465 w478] -> w380
      tunnel: w384 -> [w420 w455 w465 w478]
      tunnel: w383 -> [_ w452 _ _]
      tunnel: [w409 w451 w464 w476] -> w382
      tunnel: w381 -> [w408 w451 w464 w476]
      frame "idle", Default {
        n192 = Dequeue Element(queue=w431, timeout in ms (-1)=0) -> (element=w426:dbl, timed out?=w410:bool)  [unwired: 1 in, 2 out]
        n193 = case shown="True" w410 {
          tunnel: w426 -> [w441 _]
          tunnel: [w441 w443] -> w419
          tunnel: [w441 w445] -> w425
          tunnel: [w435 w450] -> w424
          tunnel: w423 -> [w440 w445]
          tunnel: w422 -> [w439 w450]
          tunnel: [w436 w447] -> w421
          tunnel: w420 -> [_ w447]
          tunnel: [w435 w442] -> w409
          frame False {
            n194 = call <vilib>:"High Resolution Relative Seconds.vi"() -> ("relative seconds"=w435:dbl)
            n195 = Subtract(x=w441, y=w440) -> (x-y=w438:dbl)
            n196 = Subtract(x=w435, y=w439) -> (x-y=w437:dbl)
            n197 = Divide(x=w438, y=w437) -> (x/y=w436:dbl)
          }
          frame True {
            n198 = call <vilib>:"High Resolution Relative Seconds.vi"() -> ("relative seconds"=w442:dbl)
            n199 = Subtract(x=w442, y=w450) -> (x-y=w449:dbl)
            n200 = Multiply(x=w449, y=w447) -> (x*y=w448:dbl)
            n201 = Add(x=w445, y=w448) -> (x+y=w446:dbl)
            n202 = Select(t=w446, s="interpolate output", f=w445) -> (s? t:f=w443:dbl)
          }
        }
        n203 = local read "p1 [mm]"() -> (w417:dbl)
        n204 = local read "p2 [mm]"() -> (w418:dbl)
        n205 = Subtract(x=w419, y=w417) -> (x-y=w416:dbl)
        n206 = Subtract(x=w418, y=w417) -> (x-y=w415:dbl)
        n207 = Subtract(x=w409, y=w408) -> (x-y=w407:dbl)
        n208 = Divide(x=w416, y=w415) -> (x/y=w414:dbl)
        n209 = Reciprocal(x=w407) -> ()  [unwired: 1 out]
        n210 = Multiply(x=w414, y=8.0) -> (x*y=w405:dbl)
        n211 = Increment(x=w405) -> (x+1=w404:dbl)
        "x*y" <- w404
        n212 = In Range and Coerce(upper limit=10.0, x=w404, lower limit=0.0) -> (coerced(x)=w406:dbl)  [unwired: 1 out]
        "output voltage" <- w406
        n213 = case shown="False" "Enable?" {
          tunnel: w406 -> [_ w434]
          frame False {
          }
          frame True {
            "Waveform Chart" <- w434
          }
        }
        n214 = call-poly <vilib>:"DAQmx Write.vi"("task/channels in"=w428, "data"=w406, "error in"=w427) -> ("task out"=w430:refnum<k21>, "error out"=w429:errorcluster)  [unwired: 10 in, 1 out]
      }
      frame "close" {
        n215 = Dequeue Element(queue=w463) -> (queue out=w462:refnum<queue>, error out=w461:errorcluster)  [unwired: 2 in, 2 out]
        n216 = Unbundle By Name(w452) -> ("dev2_data"=w453:refnum<queue>)
        n217 = Release Queue(queue=w462, error in (no error)=w461) -> ()  [unwired: 1 in, 3 out]
        n218 = Flush Queue(queue=w453) -> (queue out=w454:refnum<queue>)  [unwired: 1 in, 2 out]
        n219 = Release Queue(queue=w454) -> ()  [unwired: 2 in, 3 out]
      }
      frame "release" {
        n220 = Dequeue Element(queue=w474) -> ()  [unwired: 2 in, 4 out]
        n221 = call <vilib>:"DAQmx Stop Task.vi"("task/channels in"=w471, "error in"=w470) -> ("task out"=w469:refnum<k21>, "error out"=w468:errorcluster)  [unwired: 12 in]
        n222 = call <vilib>:"DAQmx Clear Task.vi"("task in"=w469, "error in"=w468) -> ("error out"=w473:errorcluster)  [unwired: 13 in]
      }
      frame "initialize" {
        w487 = -1 items=["Default"=-1, "RSE"=10083, "Differential"=10106, "Pseudodifferential"=12529] ("output terminal configuration")
        n223 = Dequeue Element(queue=w482) -> ()  [unwired: 2 in, 4 out]
        n224 = call-poly <vilib>:"DAQmx Create Virtual Channel.vi"("maximum value"=10.0, "minimum value"=0.0, "output terminal configuration"=w487, "physical channels"="physical channels", "error in"=w490) -> ("task out"=w486:refnum<k21>, "error out"=w485:errorcluster)  [unwired: 9 in]
        n225 = call <vilib>:"DAQmx Start Task.vi"("task/channels in"=w486, "error in"=w485) -> ("task out"=w484:refnum<k21>, "error out"=w483:errorcluster)  [unwired: 12 in]
      }
    }
    "meas. velocity" <- w380
    "DAC error" <- w394
  }
